vi "Build Error Cluster.vi"(1 "String to Prepend to source (\"\")":string, 2 "code":i32) -> (0 "error out":errorcluster)   [LabVIEW 2014, in "JKI State Machine++.lvlib"]
doc: "Creates an error cluster, building the source string from the calling VIs call chain in a standard LabVIEW fashon. Builds source string as:\n\"<B>Calling VI</B> in <B>Calling VI's Caller</B>-><B>Calling VI's Caller's Caller</B>->etc...->etc...\"\nOptional 'String to Prepend to source (\"\")' string input is used to add extra descriptive info to the source string. This string, if present, will be enclosed in parenthesis and prepended to the source string.\n\n<b>Inputs:</b>\n - <b>code</b>: error code\n - <b>String to Prepend to source (\"\")</b>: error string\n\n<b>Outputs:</b>\n - <b>error out</b>: Error cluster"
uses:
  JKI State Machine++.lvlib
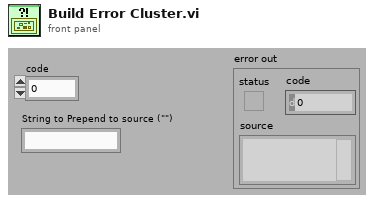
[diagram p1: front panel]
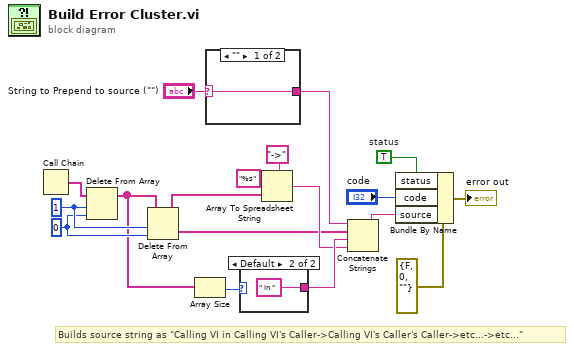
[diagram p0: block diagram]
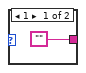
[diagram p2: hidden frame]
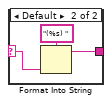
[diagram p3: hidden frame]
diagram:
  w12 = 0 ("Index")
  w13 = 1 ("Length")
  w8 = TRUE  # status
  # "Builds source string as \"Calling VI in Calling VI's Caller->Calling VI's Caller's Caller->etc...->etc...\""
  n1 = Call Chain() -> (call chain=w18:string[])
  n2 = Delete From Array(array=w18, length=w13, index=w12) -> (array with subset deleted=w1:string[])  [unwired: 1 out]
  n3 = Delete From Array(array=w1, length=w13, index=w12) -> (deleted portion=w2:string[], array with subset deleted=w11:string[])
  n4 = Array Size(array=w1) -> (size(s)=w3:i32)
  n5 = case shown="\"\"" "String to Prepend to source (\"\")" {
    selector: "String to Prepend to source (\"\")" -> [w19 w22]
    tunnel: [w19 w20] -> w4
    frame "" {
    }
    frame Default {
      n6 = Format Into String(format string="(%s) " ("Format String"), w22) -> (resulting string=w20:string)  [unwired: 2 in, 1 out]
    }
  }
  n7 = case shown="Default" w3 {
    tunnel: ["" " in " ("Format String")] -> w16
    frame 1 {
    }
    frame Default {
    }
  }
  n8 = Array To Spreadsheet String(delimiter (Tab)="->", array=w11, 3:"%s" ("format string")) -> (spreadsheet string=w15:string)
  n9 = Concatenate Strings(w4, w2, w16, w15) -> (w7:string)
  n10 = Bundle By Name(cluster=errorcluster {"status"=FALSE, "code"=0, "source"=""} ("error out"), "status"=w8, "code"="code", "source"=w7) -> (→"error out":errorcluster)
